vi "T7 Stream Config KAG-v2.vi"(0 "IP:Port":string, 5 "Stream Configuration":T2={"Scan Rate (Hz)"=1000.0, "Samples Per Packet"=512, "Resolution Index"=0, "Buffer Size (bytes)"=32768, "NumScans"=1500, "Read Timeout (ms)"=5000, "Scan Table"=[{"Channel"=0, "BipGain"=0, "Input Config"="Single-Ended"}, {"Channel"=1, "BipGain"=0, "Input Config"="Single-Ended"}, {"Channel"=2, "BipGain"=0, "Input Config"="Single-Ended"}, {"Channel"=3, "BipGain"=0, "Input Config"="Single-Ended"}]} {"Samples Per Packet" max=512 step=1; "Buffer Size (bytes)" max=32768 step=1; "Resolution Index" max=8 step=1; "Scan Rate (Hz)" max=100000; "Scan Table"."BipGain" items=["x1", "x10", "x100", "x1000"]; "Scan Table"."Channel" step=1}, 10 "STREAM Registers":T3(array[cluster])=[{"Register Num"=4990, "Register Name"="STREAM_ENABLE", "DataType"="UINT32", "Write Val"=0.0}, {"Register Num"=4002, "Register Name"="STREAM_SCANRATE_HZ", "DataType"="FLOAT32", "Write Val"=1000.0}, {"Register Num"=4004, "Register Name"="STREAM_NUM_ADDRESSES", "DataType"="UINT32", "Write Val"=4.0}, {"Register Num"=4006, "Register Name"="STREAM_SAMPLES_PER_PACKET", "DataType"="UINT32", "Write Val"=25000.0}, {"Register Num"=4008, "Register Name"="STREAM_SETTLING_US", "DataType"="FLOAT32", "Write Val"=0.0}, {"Register Num"=4010, "Register Name"="STREAM_RESOLUTION_INDEX", "DataType"="UINT32", "Write Val"=0.0}, {"Register Num"=4012, "Register Name"="STREAM_BUFFER_SIZE_BYTES", "DataType"="UINT32", "Write Val"=20000.0}, {"Register Num"=4014, "Register Name"="STREAM_OPTIONS", "DataType"="UINT32", "Write Val"=0.0}, {"Register Num"=4016, "Register Name"="STREAM_AUTO_TARGET", "DataType"="UINT32", "Write Val"=0.0}, {"Register Num"=4018, "Register Name"="STREAM_DATATYPE", "DataType"="UINT32", "Write Val"=0.0}, {"Register Num"=4020, "Register Name"="STREAM_NUM_SCANS", "DataType"="UINT32", "Write Val"=1500.0}, {"Register Num"=4022, "Register Name"="STREAM_EXTERNAL_CLOCK_DIVISOR", "DataType"="UINT32", "Write Val"=0.0}, {"Register Num"=4100, "Register Name"="STREAM_SCANLIST_ADDRESS#(0:127)", "DataType"="UINT32", "Write Val"=0.0}, {"Register Num"=4102, "Register Name"="STREAM_SCANLIST_ADDRESS#(0:127)", "DataType"="UINT32", "Write Val"=2.0}, {"Register Num"=4104, "Register Name"="STREAM_SCANLIST_ADDRESS#(0:127)", "DataType"="UINT32", "Write Val"=4.0}, {"Register Num"=4106, "Register Name"="STREAM_SCANLIST_ADDRESS#(0:127)", "DataType"="UINT32", "Write Val"=5.0}, {"Register Num"=41000, "Register Name"="AIN#(0:254)_NEGATIVE_CH", "DataType"="UINT16", "Write Val"=199.0}, {"Register Num"=41002, "Register Name"="AIN#(0:254)_NEGATIVE_CH", "DataType"="UINT16", "Write Val"=3.0}, {"Register Num"=41004, "Register Name"="AIN#(0:254)_NEGATIVE_CH", "DataType"="UINT16", "Write Val"=199.0}], 11 "error in":errorcluster) -> (6 "Strm Config Out":T2={"Scan Rate (Hz)"=1000.0, "Samples Per Packet"=512, "Resolution Index"=0, "Buffer Size (bytes)"=32768, "NumScans"=1500, "Read Timeout (ms)"=5000, "Scan Table"=[{"Channel"=0, "BipGain"=0, "Input Config"="Single-Ended"}, {"Channel"=1, "BipGain"=0, "Input Config"="Single-Ended"}, {"Channel"=2, "BipGain"=0, "Input Config"="Single-Ended"}, {"Channel"=3, "BipGain"=0, "Input Config"="Single-Ended"}]} {"Samples Per Packet" max=512 step=1; "Buffer Size (bytes)" max=32768 step=1; "Resolution Index" max=8 step=1; "Scan Rate (Hz)" max=100000; "Scan Table"."BipGain" items=["x1", "x10", "x100", "x1000"]; "Scan Table"."Channel" step=1}, 15 "error out":errorcluster)   [LabVIEW 2022 SP3]
doc: "Write Stream Configuration LabJack Registers via MODBUS. There are a set of registers which comprise the stream configuration registers, and these are written with control values for Scan Rate, NumScans, Resolution, etc. Also, the Scan Table is used to build a Scan List of Stream Configuration Registers which point to streamable AI Channels."
uses:
  T7 Stream Config KAG.ctl
  T7 Secondary Configs KAG.ctl
  T7Examples/MODBUS/T7MOD_Write_UINT16_Register.vi
  T7Examples/MODBUS/T7MOD_Write_FLOAT32_Register.vi
panel:
  in  "Secondary Stream Configurations":T1={"Settling Delay (*5 us)"=0.0, "Clock Source"=0, "Auto Target"=1} {"Auto Target" max=5000 step=1; "Clock Source" max=2 step=2; "Settling Delay (*5 us)" max=255 step=1}
  in  "Tab Control":enum32{"Stream Registers", "Stream Config Out"}(tab)
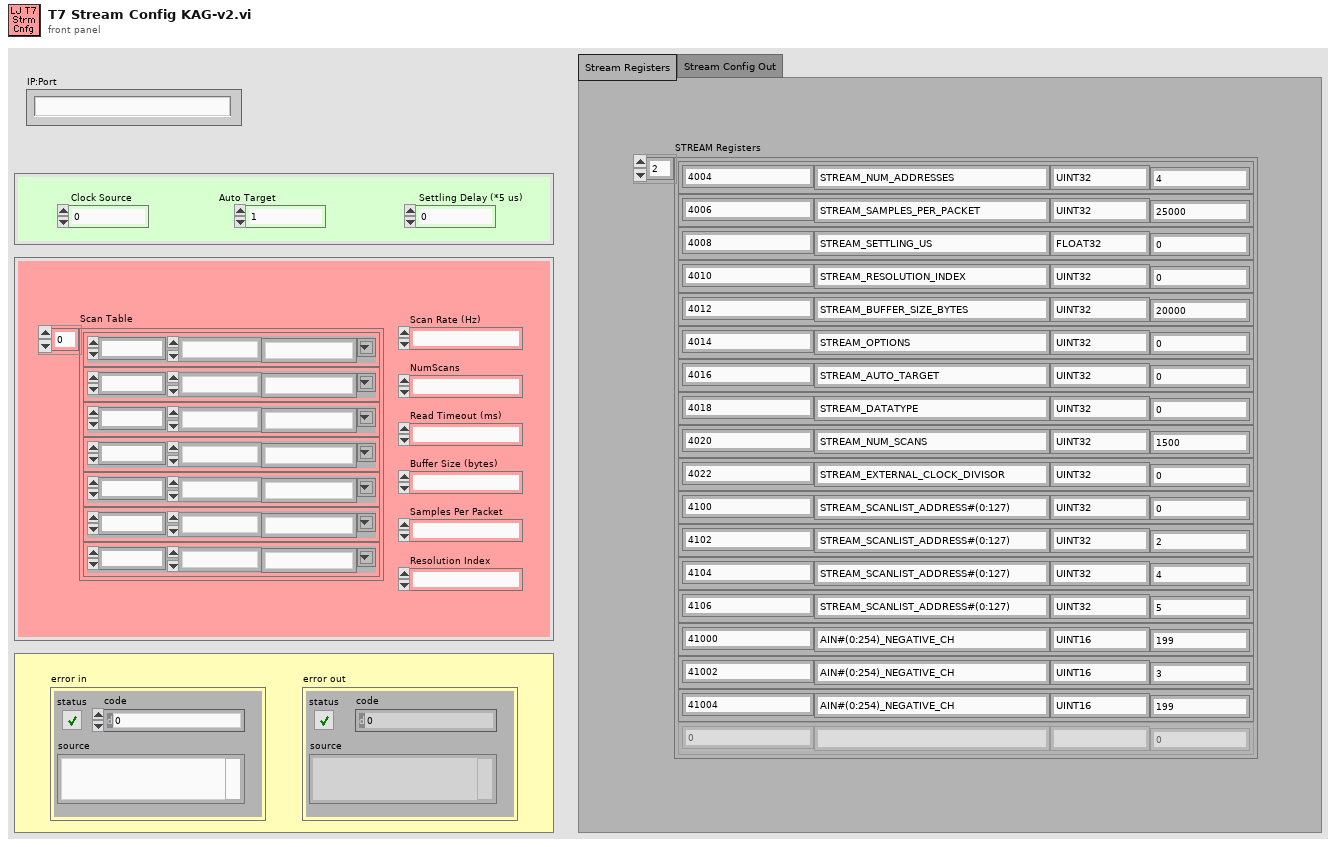
[diagram p1: front panel]
types:
  T1 = typedef "T7 Secondary Configs KAG.ctl" = cluster{"Settling Delay (*5 us)":sgl, "Clock Source":u32, "Auto Target":u32}
  T2 = typedef "T7 Stream Config KAG.ctl" = cluster{"Scan Rate (Hz)":sgl, "Samples Per Packet":u32, "Resolution Index":u32, "Buffer Size (bytes)":u32, "NumScans":u32, "Read Timeout (ms)":u32, "Scan Table":cluster{"Channel":u32, "BipGain":u32, "Input Config":string}[]}
  T3 = cluster{"Register Num":i32, "Register Name":string, "DataType":string, "Write Val":dbl}[]
  T4 = cluster{"Channel":u32, "BipGain":u32, "Input Config":string}[]
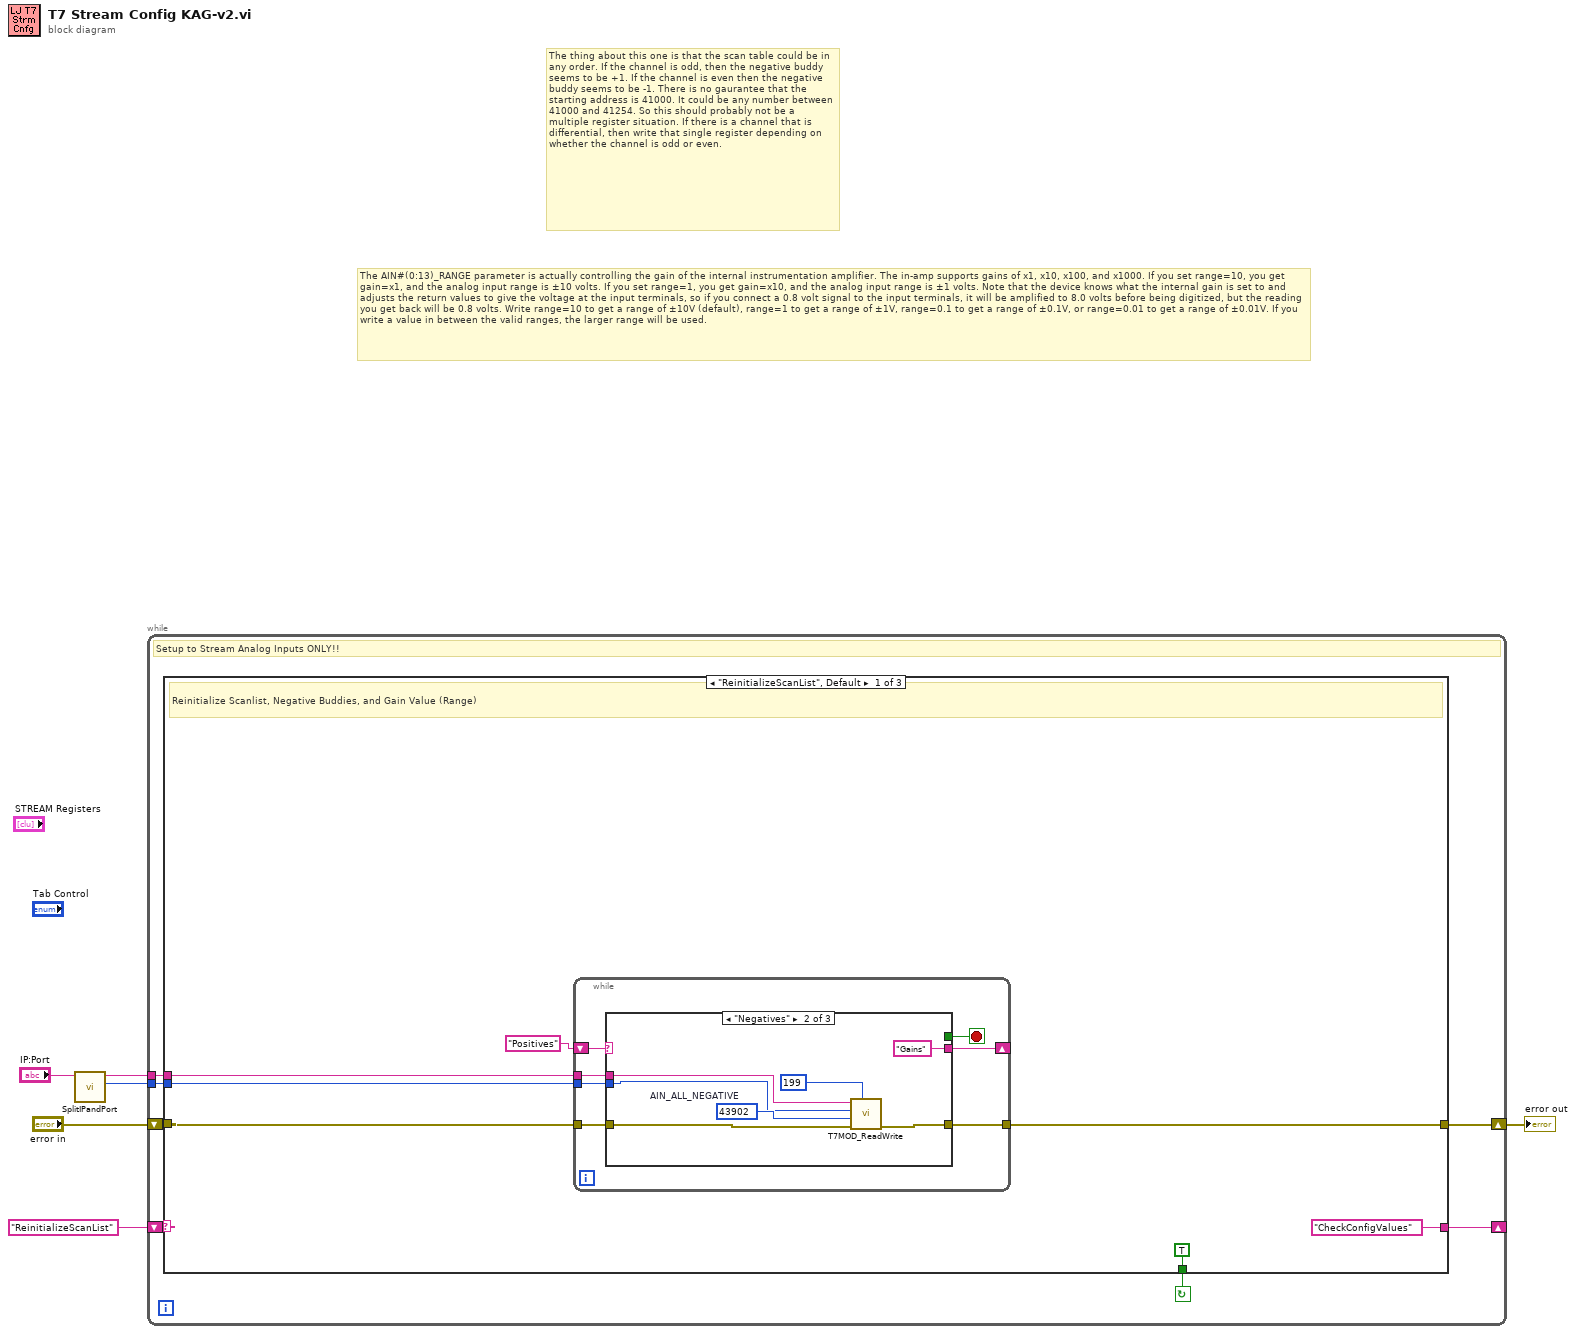
[diagram p0: block diagram]
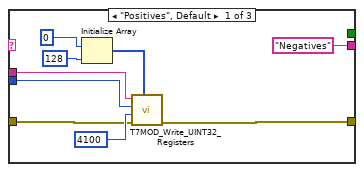
[diagram p2: hidden frame]
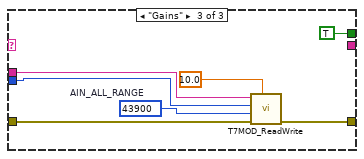
[diagram p3: hidden frame]
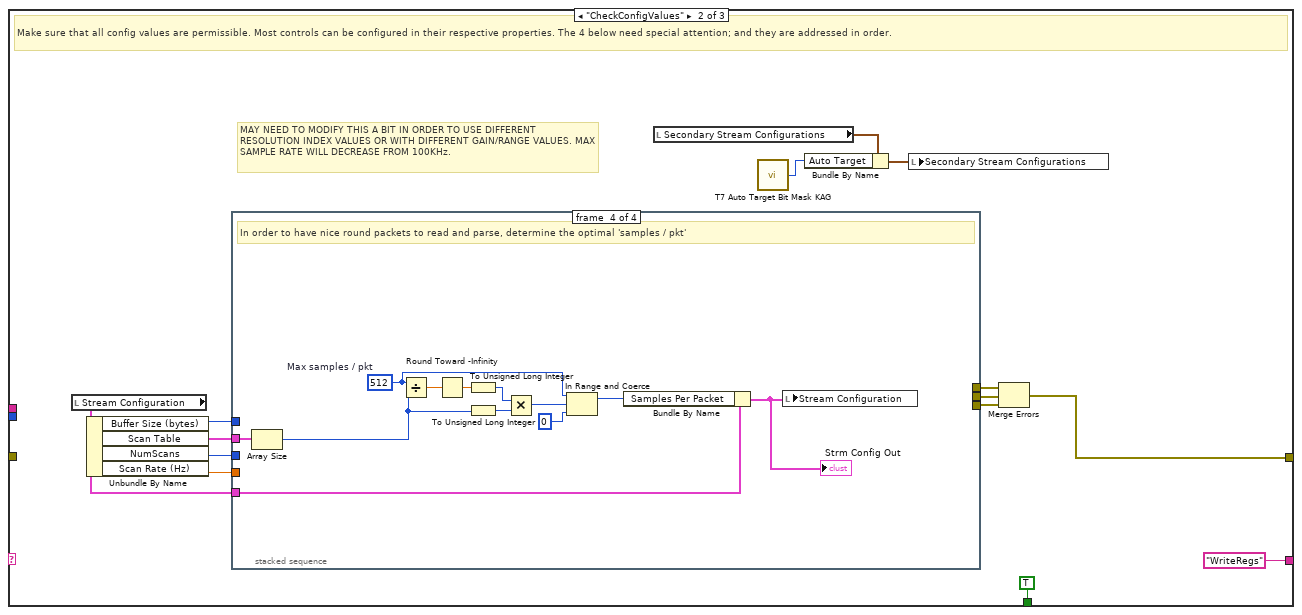
[diagram p4: hidden frame]
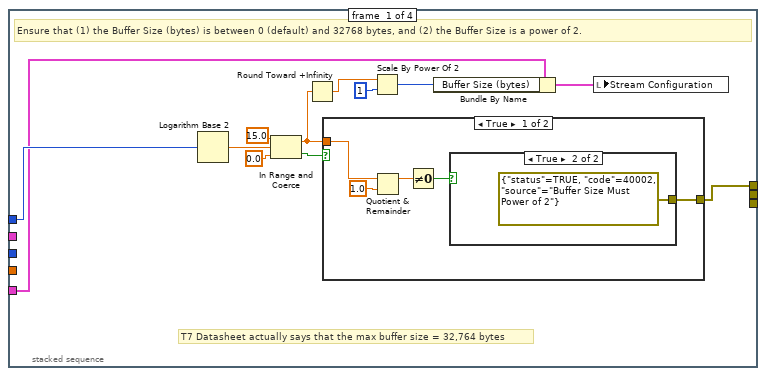
[diagram p5: hidden frame]
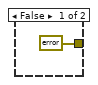
[diagram p6: hidden frame]
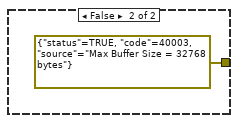
[diagram p7: hidden frame]
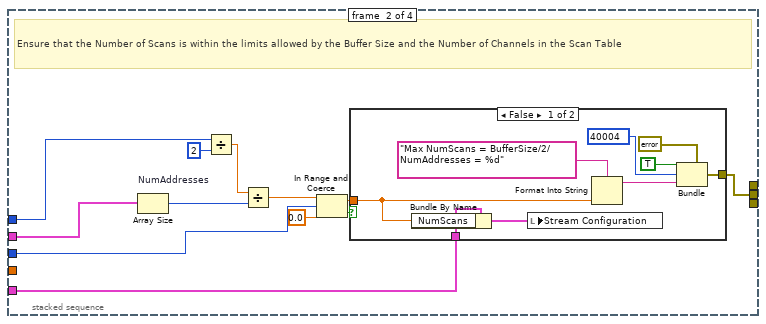
[diagram p8: hidden frame]
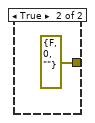
[diagram p9: hidden frame]
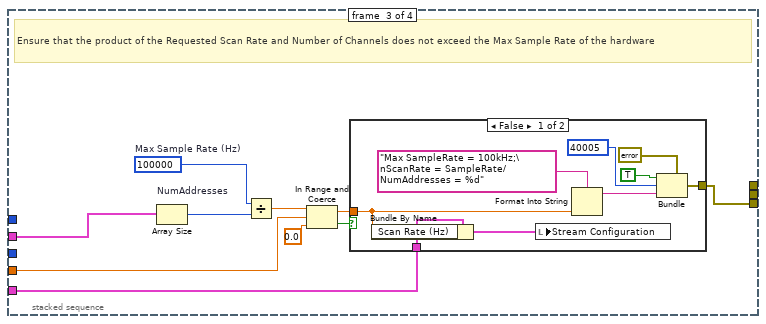
[diagram p10: hidden frame]
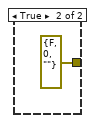
[diagram p11: hidden frame]
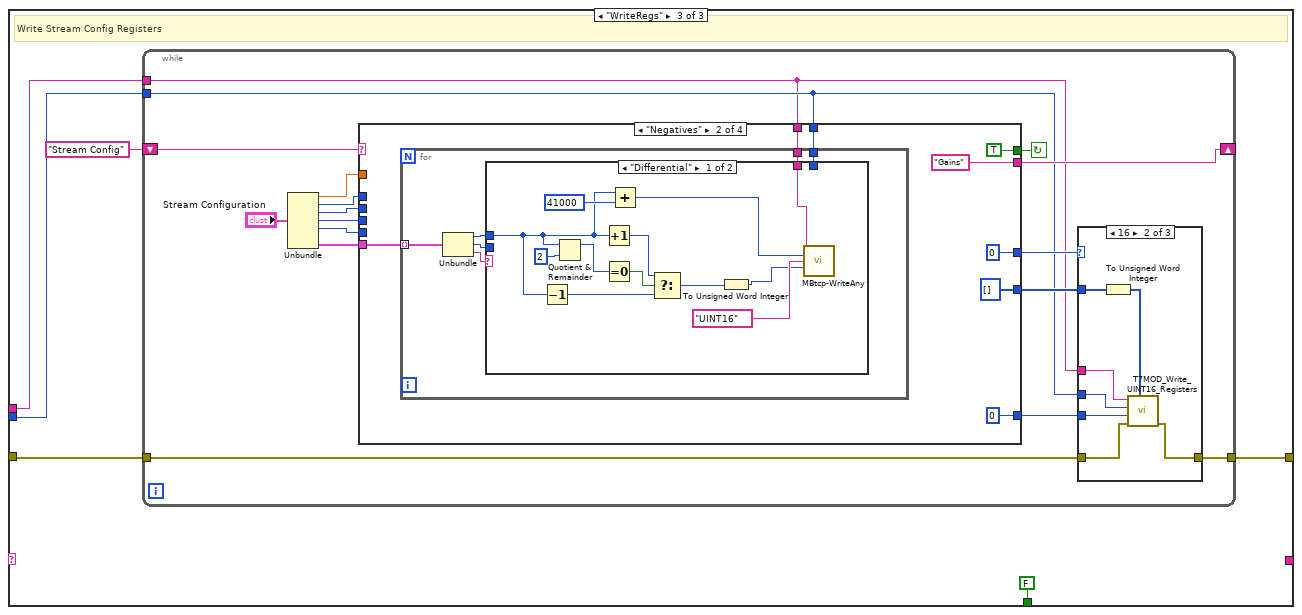
[diagram p12: hidden frame]
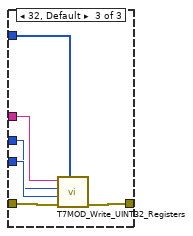
[diagram p14: hidden frame]
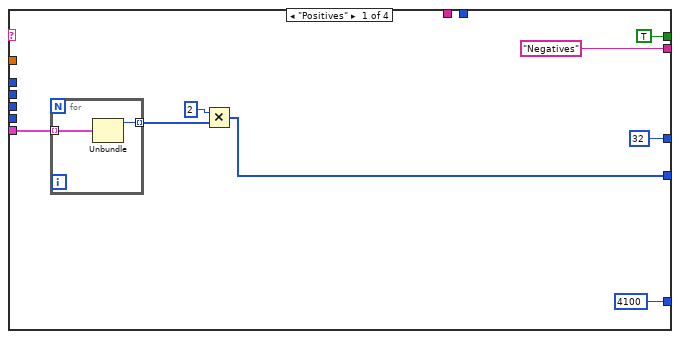
[diagram p15: hidden frame]
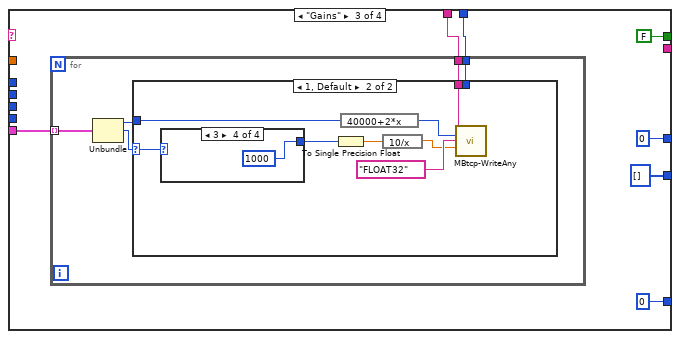
[diagram p17: hidden frame]
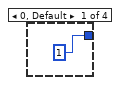
[diagram p19: hidden frame]
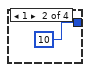
[diagram p20: hidden frame]
diagram:
  # "The AIN#(0:13)_RANGE parameter is actually controlling the gain of the internal instrumentation amplifier. The in-amp supports gains of x1, x10, x100, and x1000. If you set range=10, you get gain=x1, and the analog input range is ±10 volts. If you set range=1, you get gain=x10, and the analog input range is ±1 volts. Note that the device knows what the internal gain is set to and adjusts the return values to give the voltage at the input terminals, so if you connect a 0.8 volt signal to the input terminals, it will be amplified to 8.0 volts before being digitized, but the reading you get back will be 0.8 volts. Write range=10 to get a range of ±10V (default), range=1 to get a range of ±1V, range=0.1 to get a range of ±0.1V, or range=0.01 to get a range of ±0.01V. If you write a value in between the valid ranges, the larger range will be used."
  # "The thing about this one is that the scan table could be in any order. If the channel is odd, then the negative buddy seems to be +1. If the channel is even then the negative buddy seems to be -1. There is no gaurantee that the starting address is 41000. It could be any number between 41000 and 41254. So this should probably not be a multiple register situation. If there is a channel that is differential, then write that single register depending on whether the channel is odd or even."
  n1 = call "SplitIPandPort.vi"("IP:Port"="IP:Port") -> ("Port"=w1:u16, "IP"=w2:string)  [unwired: 9 in]
  n2 = while {
    shift-right: [w11] -> _
    shift-left: "ReinitializeScanList" -> [w13]
    shift-right: [w9] -> w4
    shift-left: "error in" -> [w10]
    tunnel: w2 -> [w8]
    tunnel: w1 -> [w7]
    stop <- w12 continue-if-true
    # "Setup to Stream Analog Inputs ONLY!!"
    n3 = case shown="\"ReinitializeScanList\", Default" w13 {
      tunnel: [TRUE TRUE FALSE] -> w12
      tunnel: ["CheckConfigValues" "WriteRegs" _] -> w11
      tunnel: w10 -> [w17 _ w142]
      tunnel: [w16 w59 w141] -> w9
      tunnel: w8 -> [w15 _ w139]
      tunnel: w7 -> [w14 _ w140]
      frame "ReinitializeScanList", Default {
        # "Reinitialize Scanlist, Negative Buddies, and Gain Value (Range)"
        n4 = while {
          shift-right: [w26] -> _
          shift-left: "Positives" -> [w27]
          tunnel: w17 -> [w24]
          tunnel: [w23] -> w16
          tunnel: w15 -> [w22]
          tunnel: w14 -> [w21]
          stop <- w25 stop-if-true
          n5 = case shown="\"Negatives\"" w27 {
            tunnel: ["Negatives" "Gains" _] -> w26
            tunnel: [_ _ TRUE] -> w25
            tunnel: w24 -> [w31 w40 w47]
            tunnel: [w30 w39 w46] -> w23
            tunnel: w22 -> [w29 w38 w45]
            tunnel: w21 -> [w28 w37 w44]
            frame "Positives", Default {
              n6 = Initialize Array(u32 0 ("UINT32 to Write"), 128) -> (w33:u32[])
              n7 = call "T7MOD_Write_UINT32_Registers.vi"("UINT32 to Write"=w33, "error in"=w31, "Starting Address"=4100, "Remote Port"=w28, "Remote IP Address"=w29) -> ("error out"=w30:errorcluster)  [unwired: 5 in, 1 out]
            }
            frame "Negatives" {
              w41 = 43902  # AIN_ALL_NEGATIVE
              n8 = call-poly "T7MOD_ReadWrite.vi"("UINT16 to Write"=u16 199 ("UINT32 to Write"), "error in"=w40, "LabJack UINT16 Register"=w41, "Remote Port"=w37, "Remote IP Address"=w38) -> ("error out"=w39:errorcluster)  [unwired: 5 in, 1 out]
            }
            frame "Gains" {
              w50 = 43900  # AIN_ALL_RANGE
              n9 = call-poly "T7MOD_ReadWrite.vi"("FLOAT32 to Write"=sgl 10.0, "error in"=w47, "LabJack FLOAT32 Register"=w50, "Remote Port"=w44, "Remote IP Address"=w45) -> ("error out"=w46:errorcluster)  [unwired: 5 in, 1 out]
            }
          }
        }
      }
      frame "CheckConfigValues" {
        # "MAY NEED TO MODIFY THIS A BIT IN ORDER TO USE DIFFERENT RESOLUTION INDEX VALUES OR WITH DIFFERENT GAIN/RANGE VALUES. MAX SAMPLE RATE WILL DECREASE FROM 100KHz."
        # "Make sure that all config values are permissible. Most controls can be configured in their respective properties. The 4 below need special attention; and they are addressed in order."
        n10 = local read "Stream Configuration"() -> (w52:T2)
        n11 = Unbundle By Name(w52) -> ("Buffer Size (bytes)"=w55:u32, "Scan Table"=w56:T4, "NumScans"=w57:u32, "Scan Rate (Hz)"=w54:sgl)
        n12 = stacked-sequence {
          tunnel: [w68 _ _ _] -> w62
          tunnel: [_ w89 _ _] -> w61
          tunnel: [_ _ w110 _] -> w60
          tunnel: w52 -> [w65 w88 w107 w134]
          tunnel: w57 -> [_ w87 _ _]
          tunnel: w56 -> [_ w86 w109 w136]
          tunnel: w55 -> [w66 w85 _ _]
          tunnel: w54 -> [_ _ w108 _]
          frame #0 {
            # "T7 Datasheet actually says that the max buffer size = 32,764 bytes"
            # "Ensure that (1) the Buffer Size (bytes) is between 0 (default) and 32768 bytes, and (2) the Buffer Size is a power of 2."
            n13 = Logarithm Base 2(1:w66) -> (0:w75:dbl)
            n14 = In Range and Coerce(upper limit=15.0 ("y"), x=w75, lower limit=0.0) -> (coerced(x)=w69:dbl, In Range?=w73:bool)
            n15 = Round Toward +Infinity(x=w69) -> (ceil(x): smallest int >= x=w71:dbl)
            n16 = case shown="True" w73 {
              tunnel: [w79 errorcluster {"status"=TRUE, "code"=40003, "source"="Max Buffer Size = 32768 bytes"} ("error constant")] -> w68
              tunnel: w69 -> [w77 _]
              frame True {
                n17 = Quotient & Remainder(x=w77, y=1.0) -> (x-y*floor(x/y)=w80:dbl)  [unwired: 1 out]
                n18 = Not Equal To 0?(x=w80) -> (x != 0?=w78:bool)
                n19 = case shown="True" w78 {
                  tunnel: [errorcluster {"status"=FALSE, "code"=0, "source"=""} ("error constant") errorcluster {"status"=TRUE, "code"=40002, "source"="Buffer Size Must Power of 2"} ("error constant")] -> w79
                  frame False {
                  }
                  frame True {
                  }
                }
              }
              frame False {
              }
            }
            n20 = Scale By Power Of 2(n=w71, x=u32 1) -> (x*2^n=w72:u32)
            n21 = Bundle By Name(cluster=w65, "Buffer Size (bytes)"=w72) -> (w67:T2)
            n22 = local write "Stream Configuration"(w67) -> ()
          }
          frame #1 {
            # "Ensure that the Number of Scans is within the limits allowed by the Buffer Size and the Number of Channels in the Scan Table"
            n23 = Array Size "NumAddresses"(array=w86) -> (size(s)=w96:i32)
            n24 = Divide(x=w85, y=u32 2) -> (x/y=w95:dbl)
            n25 = Divide(x=w95, y=w96) -> (x/y=w93:dbl)
            n26 = In Range and Coerce(upper limit=w93, x=w87, lower limit=0.0) -> (coerced(x)=w91:dbl, In Range?=w90:bool)
            n27 = case shown="False" w90 {
              tunnel: w91 -> [w99 _]
              tunnel: [w100 errorcluster {"status"=FALSE, "code"=0, "source"=""} ("error constant")] -> w89
              tunnel: w88 -> [w97 _]
              frame False {
                n28 = Bundle By Name(cluster=w97, "NumScans"=w99) -> (w98:T2)
                n29 = local write "Stream Configuration"(w98) -> ()
                n30 = Format Into String(format string="Max NumScans = BufferSize/2/NumAddresses = %d" ("initial string"), w99) -> (resulting string=w101:string)  [unwired: 2 in, 1 out]
                n31 = Bundle(cluster=errorcluster {"status"=FALSE, "code"=0, "source"=""} ("error constant"), "status"=TRUE, "code"=40004, "source"=w101) -> (w100:errorcluster)
              }
              frame True {
              }
            }
          }
          frame #2 {
            w115 = 100000  # Max Sample Rate (Hz)
            # "Ensure that the product of the Requested Scan Rate and Number of Channels does not exceed the Max Sample Rate of the hardware"
            n32 = Array Size "NumAddresses"(array=w109) -> (size(s)=w116:i32)
            n33 = Divide(x=w115, y=w116) -> (x/y=w114:dbl)
            n34 = In Range and Coerce(upper limit=w114, x=w108, lower limit=0.0) -> (coerced(x)=w111:dbl, In Range?=w112:bool)
            n35 = case shown="False" w112 {
              tunnel: w111 -> [w119 _]
              tunnel: [w120 errorcluster {"status"=FALSE, "code"=0, "source"=""} ("error constant")] -> w110
              tunnel: w107 -> [w117 _]
              frame False {
                n36 = Bundle By Name(cluster=w117, "Scan Rate (Hz)"=w119) -> (w118:T2)
                n37 = local write "Stream Configuration"(w118) -> ()
                n38 = Format Into String(format string="Max SampleRate = 100kHz;\nScanRate = SampleRate/NumAddresses = %d" ("initial string"), w119) -> (resulting string=w121:string)  [unwired: 2 in, 1 out]
                n39 = Bundle(cluster=errorcluster {"status"=FALSE, "code"=0, "source"=""} ("error constant"), "status"=TRUE, "code"=40005, "source"=w121) -> (w120:errorcluster)
              }
              frame True {
              }
            }
          }
          frame #3 {
            w129 = 512  # Max samples / pkt
            # "In order to have nice round packets to read and parse, determine the optimal 'samples / pkt'"
            n40 = Array Size(array=w136) -> (size(s)=w135:i32)
            n41 = Divide(x=w129, y=w135) -> (x/y=w138:dbl)
            n42 = Round Toward -Infinity(1:w138) -> (0:w137:dbl)
            n43 = To Unsigned Long Integer(number=w137) -> (unsigned 32bit integer=w133:u32)
            n44 = To Unsigned Long Integer(number=w135) -> (unsigned 32bit integer=w132:u32)
            n45 = Multiply(x=w133, y=w132) -> (x*y=w131:u32)
            n46 = In Range and Coerce(upper limit=w129, x=w131, lower limit=u32 0) -> (coerced(x)=w128:u32)  [unwired: 1 out]
            n47 = Bundle By Name(cluster=w134, "Samples Per Packet"=w128) -> (w127:T2)
            "Strm Config Out" <- w127
            n48 = local write "Stream Configuration"(w127) -> ()
          }
        }
        n49 = local read "Secondary Stream Configurations"() -> (w51:T1)
        n50 = call "T7 Auto Target Bit Mask KAG.vi"() -> ("Auto Target"=w58:u32)  [unwired: 1 in]
        n51 = Bundle By Name(cluster=w51, "Auto Target"=w58) -> (w53:T1)
        n52 = local write "Secondary Stream Configurations"(w53) -> ()
        n53 = Merge Errors(w62, w61, w60) -> (w59:errorcluster)
      }
      frame "WriteRegs" {
        # "Write Stream Config Registers"
        n54 = while {
          shift-right: [w147] -> _
          shift-left: "Stream Config" -> [w152]
          tunnel: w142 -> [w150]
          tunnel: [w149] -> w141
          tunnel: w140 -> [w146]
          tunnel: w139 -> [w145]
          stop <- w148 continue-if-true
          n55 = Unbundle("Stream Configuration") -> ("Scan Rate (Hz)"=w157:sgl, "Samples Per Packet"=w156:u32, "Resolution Index"=w155:u32, "Buffer Size (bytes)"=w154:u32, "NumScans"=w153:u32, "Scan Table"=w158:T4)  [unwired: 1 out]
          n56 = case shown="\"Negatives\"" w152 {
            tunnel: [4100 ("Starting Address") 0 ("Starting Address") 0 ("Starting Address") 4002 ("Starting Address")] -> w161
            tunnel: [w180 u32[] [] u32[] [] w245] -> w160
            tunnel: w158 -> [w179 w193 w218 w239]
            tunnel: w157 -> [_ _ _ w244]
            tunnel: w156 -> [_ _ _ w243]
            tunnel: w155 -> [_ _ _ w242]
            tunnel: w154 -> [_ _ _ w241]
            tunnel: w153 -> [_ _ _ w240]
            tunnel: [32 0 0 32] -> w151
            tunnel: [TRUE TRUE FALSE TRUE] -> w148
            tunnel: ["Negatives" "Gains" _ "Positives"] -> w147
            tunnel: w146 -> [_ w187 w213 _]
            tunnel: w145 -> [_ w186 w212 _]
            frame "Positives" {
              n57 = for {
                tunnel: w179 -> [w185] mode=indexing
                tunnel: [w184] -> w182 mode=indexing
                n58 = Unbundle(w185) -> ("Channel"=w184:u32)  [unwired: 2 out]
              }
              n59 = Multiply(x=u32 2, y=w182) -> (x*y=w180:u32[])
            }
            frame "Negatives" {
              n60 = for {
                tunnel: w193 -> [w199] mode=indexing
                tunnel: w187 -> [w195]
                tunnel: w186 -> [w194]
                n61 = Unbundle(w199) -> ("Channel"=w197:u32, "BipGain"=w196:u32, "Input Config"=w198:string)
                n62 = case shown="\"Differential\"" w198 {
                  tunnel: w197 -> [w204 _]
                  tunnel: w196 -> [_ _]
                  tunnel: w195 -> [_ _]
                  tunnel: w194 -> [w202 _]
                  frame "Differential" {
                    n63 = Decrement(x=w204) -> (x-1=w209:u32)
                    n64 = Quotient & Remainder(x=w204, y=u32 2) -> (x-y*floor(x/y)=w206:u32)  [unwired: 1 out]
                    n65 = Increment(x=w204) -> (x+1=w210:u32)
                    n66 = Equal To 0?(x=w206) -> (x = 0?=w211:bool)
                    n67 = Add(x=w204, y=41000 ("Starting Address")) -> (x+y=w203:u32)
                    n68 = Select(t=w210, s=w211, f=w209) -> (s? t:f=w208:u32)
                    n69 = To Unsigned Word Integer(number=w208) -> (unsigned 16bit integer=w200:u16)
                    n70 = call "MBtcp-WriteAny.vi"("IP Address"=w202, "Register"=w203, "DataType(:RegisterType)"="UINT16" ("Data type"), "Value to Output"=w200) -> ()  [unwired: 11 in, 1 out]
                  }
                  frame "Single-Ended", Default {
                  }
                }
              }
            }
            frame "Gains" {
              n71 = for {
                tunnel: w218 -> [w223] mode=indexing
                tunnel: w213 -> [w220]
                tunnel: w212 -> [w219]
                n72 = Unbundle(w223) -> ("Channel"=w221:u32, "BipGain"=w222:u32)  [unwired: 1 out]
                n73 = case shown="1, Default" w222 {
                  selector: w222 -> [_ w229]
                  tunnel: w221 -> [_ w231]
                  tunnel: w220 -> [_ _]
                  tunnel: w219 -> [_ w226]
                  frame 0 {
                  }
                  frame 1, Default {
                    n74 = case shown="3" w229 {
                      tunnel: [1 10 100 1000] -> w228
                      frame 0, Default {
                      }
                      frame 1 {
                      }
                      frame 2 {
                      }
                      frame 3 {
                      }
                    }
                    n75 = To Single Precision Float(number=w228) -> (single precision float=w230:sgl)
                    n76 = expression code="40000+2*x"(w231) -> (w227:u32)
                    n77 = expression code="10/x"(w230) -> (w224:sgl)
                    n78 = call "MBtcp-WriteAny.vi"("IP Address"=w226, "Register"=w227, "DataType(:RegisterType)"="FLOAT32" ("Data type"), "Value to Output"=w224) -> ()  [unwired: 11 in, 1 out]
                  }
                }
              }
            }
            frame "Stream Config", Default {
              w247 = u32 0
              w257 = u32 0
              n79 = Array Size "Num Addresses"(array=w239) -> (size(s)=w255:i32)
              n80 = disable-structure shown="Enabled" {
                disable-tunnel: [w258 u32 0 ("NumScans")] -> w256
                disable-tunnel: w240 -> [w258 _]
                frame Disabled {
                }
                frame Enabled {
                }
              }
              n81 = To Unsigned Long Integer(number=w255) -> (unsigned 32bit integer=w249:u32)
              n82 = Unbundle("Secondary Stream Configurations") -> ("Settling Delay (*5 us)"=w253:sgl, "Clock Source"=w252:u32, "Auto Target"=w251:u32)
              n83 = Type Cast(type=w247, x=w244) -> (*(type *) &x=w250:u32)
              n84 = Type Cast(type=w247, x=w253) -> (*(type *) &x=w248:u32)
              n85 = Build Array(w250, w249, w243, w248, w242, w241, w252, w251, w257, w256, w257) -> (w245:u32[])
            }
          }
          n86 = case shown="16" w151 {
            tunnel: w161 -> [_ w166 w175]
            tunnel: w160 -> [_ w169 w174]
            tunnel: w145 -> [_ w168 w173]
            tunnel: w146 -> [_ w167 w172]
            tunnel: w150 -> [w162 w165 w171]
            tunnel: [w162 w164 w170] -> w149
            frame 0 {
            }
            frame 16 {
              n87 = To Unsigned Word Integer(number=w169) -> (unsigned 16bit integer=w163:u16[])
              n88 = call "T7MOD_Write_UINT16_Registers.vi"("UINT16 to Write"=w163, "error in"=w165, "Starting Address"=w166, "Remote Port"=w167, "Remote IP Address"=w168) -> ("error out"=w164:errorcluster)  [unwired: 5 in, 1 out]
            }
            frame 32, Default {
              n89 = call "T7MOD_Write_UINT32_Registers.vi"("UINT32 to Write"=w174, "error in"=w171, "Starting Address"=w175, "Remote Port"=w172, "Remote IP Address"=w173) -> ("error out"=w170:errorcluster)  [unwired: 5 in, 1 out]
            }
          }
        }
      }
    }
  }
  "error out" <- w4
